vi "Check Dependent Logs.vi"(8 "error in (no error)":errorcluster, 10 "Dependent Logs":i32[](array[numeric]), 11 "Log Queues in":T1[](array[typedef])) -> (0 "error out":errorcluster, 2 "Active":bool, 3 "Log Queues out":T1[](array[typedef]))   [LabVIEW 2012, in "Waveform Data Logger Engine.lvlib"]
uses:
  Waveform Data Logger Engine.lvlib
  Types/Log Queues.ctl
  Types/Log Status.ctl
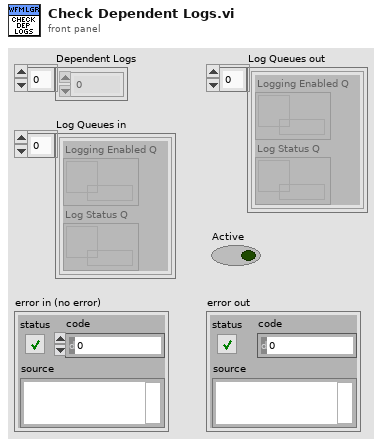
[diagram p1: front panel]
types:
  T1 = typedef "Waveform Data Logger Engine.lvlib/Log Queues.ctl" = cluster{"Logging Enabled Q":refnum<queue>, "Log Status Q":refnum<queue>}
  T2 = typedef "Waveform Data Logger Engine.lvlib/Log Status.ctl" = cluster{"Open Instances":i32, "Active Instances":i32, "Missed Samples":u64, "Error Code":i32}
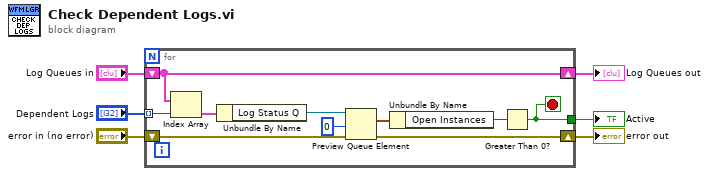
[diagram p0: block diagram]
diagram:
  n1 = for {
    tunnel: "Dependent Logs" -> [w16] mode=indexing
    shift-right: [w11] -> w6
    shift-left: "error in (no error)" -> [w13]
    shift-right: [w10] -> w4
    shift-left: "Log Queues in" -> [w10]
    tunnel: [w7] -> w5
    stop <- w7 stop-if-true
    n2 = Index Array(array=w10, index=w16) -> (element=w15:T1)
    n3 = Unbundle By Name(w15) -> ("Log Status Q"=w14:refnum<queue>)
    n4 = Preview Queue Element(queue=w14, timeout in ms (-1)=0, error in (no error)=w13) -> (element=w9:T2, error out=w11:errorcluster)  [unwired: 2 out]
    n5 = Unbundle By Name(w9) -> ("Open Instances"=w8:i32)
    n6 = Greater Than 0?(x=w8) -> (x > 0?=w7:bool)
  }
  "error out" <- w6
  "Active" <- w5
  "Log Queues out" <- w4
